vi "AES-Cipher-text.vi"(5 "Initializer Vector":string, 7 "Operation Mode":T1, 8 "error in (no error)":errorcluster, 10 "Cipher Key":string, 11 "Message in":string) -> (0 "error out":errorcluster, 3 "Ciphered message":string)   [LabVIEW 2010, in "Encryption.lvlib"]
doc: "Encripts the <b>text<b> in using the cipher and the given <b>Operation Mode</b>.\nCAUTION:\nThis VI is not secure, it does not protect the memory of the encryption, key and unencrypted data.\n\n(c) Ton Plomp, 2011\nTHIS SOFTWARE IS PROVIDED AS IS, AND ANY WARRANTY IS REJECTED"
uses:
  Encryption.lvlib
  AES-Modes.ctl
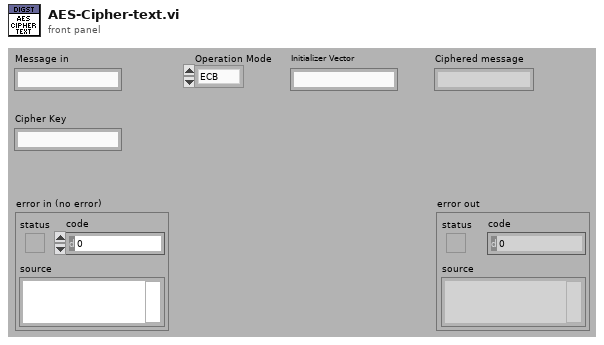
[diagram p1: front panel]
types:
  T1 = typedef "Encryption.lvlib/AES-Modes.ctl" = enum16{"ECB", "CBC", "CFB128", "OFB"}
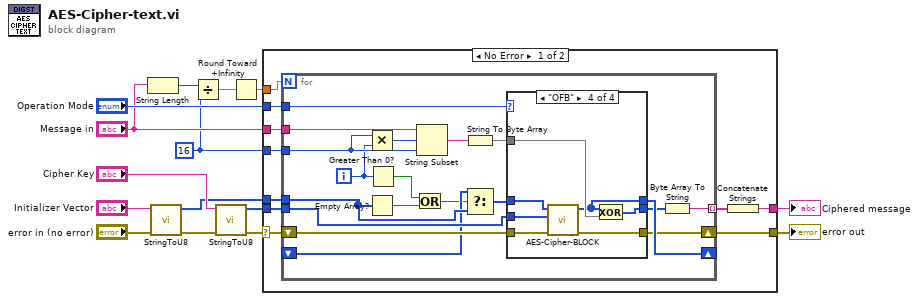
[diagram p0: block diagram]
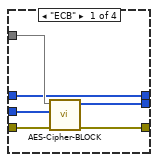
[diagram p2: hidden frame]
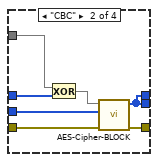
[diagram p3: hidden frame]
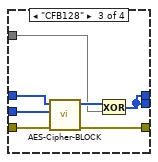
[diagram p4: hidden frame]
diagram:
  w1 = 16 ("y")
  n1 = String Length(string="Message in") -> (length=w2:i32)
  n2 = call "StringToU8.vi"("error in (no error)"="error in (no error)", "HEX text in"="Initializer Vector") -> ("error out"=w8:errorcluster, "ArrayU8 out"=w6:u8[])  [unwired: 8 in]
  n3 = Divide(x=w2, y=w1) -> (x/y=w4:dbl)
  n4 = call "StringToU8.vi"("error in (no error)"=w8, "HEX text in"="Cipher Key") -> ("error out"=w13:errorcluster, "ArrayU8 out"=w12:u8[])  [unwired: 8 in]
  n5 = Round Toward +Infinity(x=w4) -> (ceil(x): smallest int >= x=w3:dbl)
  n6 = case shown="No Error" w13 {
    selector: w13 -> [w21 w72]
    tunnel: "Message in" -> [w25 _]
    tunnel: [w20 w72] -> w15
    tunnel: w12 -> [w24 _]
    tunnel: w3 -> [w23 _]
    tunnel: w1 -> [w22 _]
    tunnel: [w18 _] -> w11
    tunnel: "Operation Mode" -> [w17 _]
    tunnel: w6 -> [w16 _]
    frame No Error {
      n7 = for {
        N: w23 -> [_]
        tunnel: w25 -> [w36]
        tunnel: w24 -> [w44]
        tunnel: w22 -> [w42]
        shift-right: [w28] -> w20
        shift-left: w21 -> [w39]
        tunnel: [w27] -> w19 mode=indexing
        tunnel: w17 -> [w38]
        shift-right: [w37] -> _
        shift-left: _ -> [w33]
        tunnel: w16 -> [w35]
        i -> [w31]
        n8 = Multiply(x=w42, y=w31) -> (x*y=w43:i32)
        n9 = Empty Array?(array=w35) -> (empty?=w30:bool)
        n10 = Greater Than 0?(x=w31) -> (x > 0?=w32:bool)
        n11 = Or(x=w32, y=w30) -> (x .or. y?=w29:bool)
        n12 = String Subset(string=w36, offset (0)=w43, length (rest)=w42) -> (substring=w41:string)
        n13 = String To Byte Array(string=w41) -> (unsigned byte array=w40:u8[])
        n14 = Select(t=w33, s=w29, f=w35) -> (s? t:f=w34:u8[])
        n15 = case shown="\"OFB\"" w38 {
          tunnel: w44 -> [w50 w57 w64 w71]
          tunnel: w40 -> [w49 w51 w59 w67]
          tunnel: w39 -> [w48 w56 w63 w70]
          tunnel: [w47 w53 w58 w66] -> w26
          tunnel: [w46 w55 w62 w69] -> w28
          tunnel: w34 -> [w45 w54 w61 w68]
          tunnel: [w45 w53 w58 w65] -> w37
          frame "ECB" {
            n16 = call "AES-Cipher-BLOCK.vi"("error in (no error)"=w48, "Cipher Key"=w50, "Plain [U8]"=w49) -> ("error out"=w46:errorcluster, "cipher [U8]"=w47:u8[])  [unwired: 7 in]
          }
          frame "CBC" {
            n17 = Exclusive Or(1:w54, 2:w51) -> (0:w52:u8[])
            n18 = call "AES-Cipher-BLOCK.vi"("error in (no error)"=w56, "Cipher Key"=w57, "Plain [U8]"=w52) -> ("error out"=w55:errorcluster, "cipher [U8]"=w53:u8[])  [unwired: 7 in]
          }
          frame "CFB128" {
            n19 = call "AES-Cipher-BLOCK.vi"("error in (no error)"=w63, "Cipher Key"=w64, "Plain [U8]"=w61) -> ("error out"=w62:errorcluster, "cipher [U8]"=w60:u8[])  [unwired: 7 in]
            n20 = Exclusive Or(1:w59, 2:w60) -> (0:w58:u8[])
          }
          frame "OFB" {
            n21 = call "AES-Cipher-BLOCK.vi"("error in (no error)"=w70, "Cipher Key"=w71, "Plain [U8]"=w68) -> ("error out"=w69:errorcluster, "cipher [U8]"=w65:u8[])  [unwired: 7 in]
            n22 = Exclusive Or(1:w67, 2:w65) -> (0:w66:u8[])
          }
        }
        n23 = Byte Array To String(unsigned byte array=w26) -> (string=w27:string)
      }
      n24 = Concatenate Strings(w19) -> (w18:string)
    }
    frame Error {
    }
  }
  "error out" <- w15
  "Ciphered message" <- w11
